vi "ShowBead.vi"(2 "save images to new location":bool, 3 "destination":path=path "H:/data/images/movies/loop around magnetic bead") -> (0 "ImageplusRois":u8[][](graph), 1 "image size":i32[](array[numeric]))   [LabVIEW 2011]
uses:
  <vilib>/vision/NI_Vision_Development_Module.lvlib
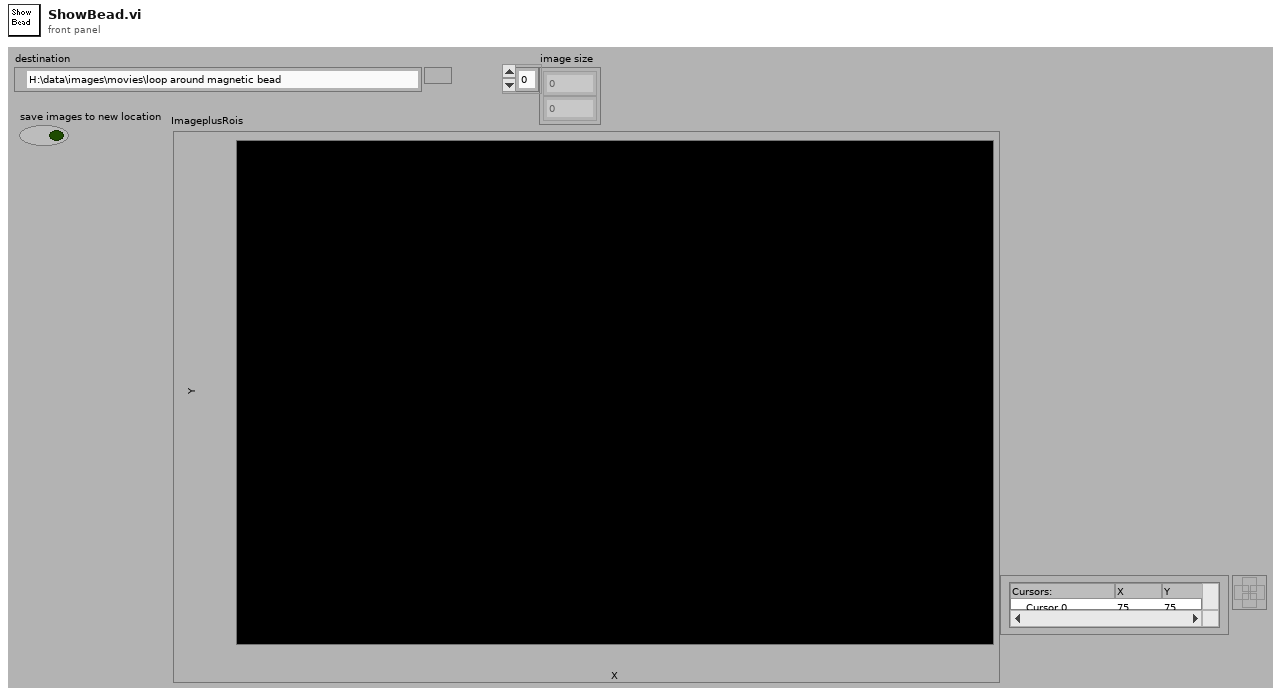
[diagram p1: front panel]
types:
  T1 = typedef "IMAQ Image.ctl" = refnum<image>
  T2 = cluster{"front panel settings":cluster{"files":cluster{"LUT path":path, "Trace path":path, " folders #":i32, "base path":path, "use trace":bool, "use base":bool, "LUT tmp":i32, "Trace tmp":i32, "active path":path}, "Tracking":cluster{"RminZ (pix)":i32, "Rmax (pix)":i32, "angular pixel \ncoverage factor":dbl, "radial pixel \ncoverage factor":dbl}, "Frames":cluster{"Start frame":i32, "number of frames":u32, "display frame ":i32, "track every nd frame ":i32, "Track all frames":bool, "active frame":i32}, "Calibs":cluster{"Zlut number of steps":i32, "pix/um":dbl, "Z correction factor":dbl, "Zlut step size (um)":dbl, "ROI(pix)":i32}, "Beads":cluster{"number of ref beads":i32, "overlay":bool}, "Misc":cluster{"save images to new location":bool, "destination":path}}, "data":cluster{"Image":T1, "image size":i32[], "Bead Array":i32[][], "overlay image":T1, "# beads":i32, "Job list":string[][], "job running":bool, "job #":i32, "folders to go":i32}}
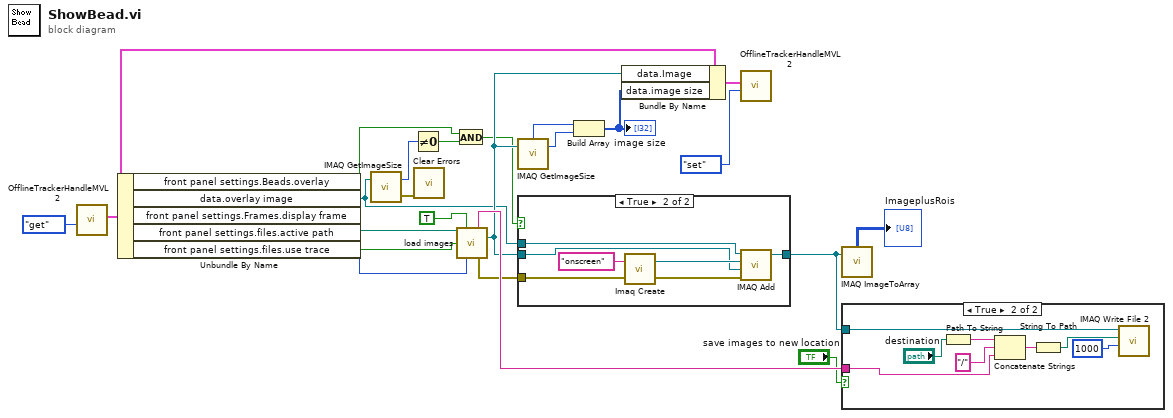
[diagram p0: block diagram]
diagram:
  n1 = call "OfflineTrackerHandleMVL2.vi"("action"=enum16{"get", "set"}."get") -> ("out"=w11:T2)  [unwired: 5 in, 1 out]
  n2 = Unbundle By Name(w11) -> ("front panel settings.Beads.overlay"=w3:bool, "data.overlay image"=w6:T1, "front panel settings.Frames.display frame"=w14:i32, "front panel settings.files.active path"=w7:path, "front panel settings.files.use trace"=w13:bool)
  n3 = call "IMAQ GetImageSize"("Image"=w6) -> ("Y Resolution"=w4:i32, "error out"=w5:errorcluster)  [unwired: 3 in, 1 out]
  n4 = Not Equal To 0?(x=w4) -> (x != 0?=w1:bool)
  n5 = call <vilib>:"Clear Errors.vi"("error in (no error)"=w5) -> ()  [unwired: 6 in, 1 out]
  n6 = And(x=w3, y=w1) -> (x .and. y?=w2:bool)
  n7 = call "load images.vi"("selected data path"=w7, "DataMarijnFormat"=TRUE, "Data(T)orLUT(F)?"=w13, "frame no."=w14) -> ("image name"=w23:string, "Image Out"=w9:T1, "error out"=w21:errorcluster)  [unwired: 2 in, 7 out]
  n8 = call "IMAQ GetImageSize"("Image"=w9) -> ("Y Resolution"=w19:i32, "X Resolution"=w20:i32)  [unwired: 1 in, 3 out]
  n9 = case shown="True" w2 {
    tunnel: w21 -> [_ w29]
    tunnel: w9 -> [w24 w27]
    tunnel: w6 -> [_ w26]
    tunnel: [w24 w25] -> w18
    frame False {
    }
    frame True {
      n10 = call "Imaq Create"("Image Name"="onscreen", "error in (no error)"=w29) -> ("New Image"=w31:T1, "error out"=w28:errorcluster)  [unwired: 2 in, 1 out]
      n11 = call "IMAQ Add"("Image Src A"=w26, "Image Dst"=w31, "Image Src B"=w27, "error in (no error)"=w28) -> ("Image Dst Out"=w25:T1)  [unwired: 1 in, 3 out]
    }
  }
  n12 = Build Array(w20, w19) -> (w10:i32[])
  "image size" <- w10
  n13 = Bundle By Name(cluster=w11, "data.Image"=w9, "data.image size"=w10) -> (w8:T2)
  n14 = call "OfflineTrackerHandleMVL2.vi"("action"=enum16{"get", "set"}."set", "in"=w8) -> ()  [unwired: 4 in, 2 out]
  n15 = call "IMAQ ImageToArray"("Image"=w18) -> ("Image Pixels (U8)"=→"ImageplusRois":u8[][])  [unwired: 2 in, 5 out]
  n16 = case shown="True" "save images to new location" {
    tunnel: w18 -> [_ w39]
    tunnel: w23 -> [_ w32]
    frame False {
    }
    frame True {
      n17 = Path To String(path="destination") -> (string=w34:string)
      n18 = Concatenate Strings(w34, "/" ("string"), w32) -> (w36:string)
      n19 = String To Path(string=w36) -> (path=w35:path)
      n20 = call-poly "IMAQ Write File 2"("Image Quality"=u32 1000, "File Path"=w35, "Image"=w39) -> ()  [unwired: 2 in, 7 out]
    }
  }
